vi "Begin.vi"(8 "error in":errorcluster) -> (0 "error out":errorcluster)   [LabVIEW 2014]
doc: "Called before other user functions, this VI is expected to open initial I/O refnums, load in file data, and do all program initialization. Notice that the <B>error out</B> terminal is simply used for data flow. Wiring it to other structures or subVIs ensures that this VI runs first."
uses:
  <vilib>/Rock Robotics/WPI/DriverStation/WPI_DriverStationRobotMode2.ctl
  <vilib>/Rock Robotics/WPI/Joystick/WPI_JoystickDeviceEnum.ctl
  <vilib>/Rock Robotics/SystemInterfaces/DIO/FPGA_DIOChannel.ctl
  <vilib>/Rock Robotics/WPI/Encoder/WPI_EncoderType.ctl
  <vilib>/Rock Robotics/WPI/Solenoid/WPI_SolenoidChannel.ctl
  <vilib>/Rock Robotics/SystemInterfaces/Typedef/FPGA_TypedefDigitalModule.ctl
  <vilib>/Rock Robotics/SystemInterfaces/Typedef/FPGA_TypedefAnalogModuleForGyro.ctl
  <vilib>/Rock Robotics/SystemInterfaces/AI/FPGA_AIGyroChannel.ctl
  <vilib>/Rock Robotics/WPI/SafetyOutput/WPI_SafetyOutputConfigMenu.ctl
  Robot Global Data.vi
  <vilib>/Rock Robotics/Network Tables/SD Write String Array.vi
  <vilib>/Rock Robotics/WPI/Counter/WPI_CounterDigitalInputToDigitalSource.vi
  <vilib>/Rock Robotics/WPI/Solenoid/WPI_SolenoidOpenDouble.vi
  <vilib>/Rock Robotics/WPI/Compressor/WPI_CompressorGetSetRefNum.vi
  <vilib>/Rock Robotics/WPI/MotorControl/WPI_MotorControlOpenCANTalonSRX.vi
  <vilib>/Rock Robotics/WPI/RobotDrive/WPI_RobotDriveOpen2MotorWithCANTalonSRX.vi
  <vilib>/Rock Robotics/SystemInterfaces/DIO/FPGA_DIOPWMChannel.ctl
  <vilib>/Rock Robotics/WPI/MotorControl/WPI_MotorControlOpen Talon.vi
  <vilib>/Rock Robotics/SystemInterfaces/i2clib/i2c_bus.ctl
  <vilib>/Rock Robotics/WPI/RobotDrive/WPI_RobotDriveOpen4MotorWithCANTalonSRX.vi
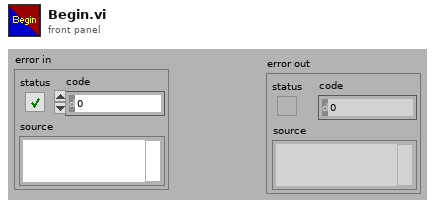
[diagram p1: front panel]
types:
  T1 = typedef "WPI_JoystickDeviceEnum.ctl" = enum16{"USB 0", "USB 1", "USB 2", "USB 3", "USB 4", "USB 5"}
  T2 = typedef "FPGA_DIOChannel.ctl" = enum8{"DIO 0", "DIO 1", "DIO 2", "DIO 3", "DIO 4", "DIO 5", "DIO 6", "DIO 7", "DIO 8", "DIO 9", "DIO MXP 0", "DIO MXP 1", "DIO MXP 2", "DIO MXP 3", "DIO MXP 4", "DIO MXP 5", "DIO MXP 6", "DIO MXP 7", "DIO MXP 8", "DIO MXP 9", "DIO MXP 10", "DIO MXP 11", "DIO MXP 12", "DIO MXP 13", "DIO MXP 14", "DIO MXP 15", "Invalid"}
  T3 = typedef "WPI_SolenoidChannel.ctl" = enum8{"Solenoid 0", "Solenoid 1", "Solenoid 2", "Solenoid 3", "Solenoid 4", "Solenoid 5", "Solenoid 6", "Solenoid 7", "Invalid"}
  T4 = typedef "FPGA_TypedefDigitalModule.ctl" = enum16{"Controller 1"}
  T5 = typedef "FPGA_AIGyroChannel.ctl" = enum8{"AI 0", "AI 1", "Invalid"}
  T6 = typedef "FPGA_TypedefAnalogModuleForGyro.ctl" = enum16{"Controller 1"}
  T7 = typedef "WPI_EncoderType.ctl" = enum16{"1x", "2x", "4x"}
  T8 = typedef "WPI_DriverStationRobotMode2.ctl" = enum16{"Autonomous Disabled", "Autonomous Enabled", "Teleop Disabled", "Teleop Enabled", "Disconnected", "Finish", "Test Disabled", "Test Enabled", "Emergency Stopped"}
  T9 = typedef "WPI_JoystickDevRef.ctl" = cluster{"Device":T1}
  T10 = typedef "WPI_CompressorDevRef.ctl" = cluster{"DevStatus":errorcluster, "Pneumatics Control Module":u8}
  T11 = typedef "WPI_SafetyOutputConfigMenu.ctl" = enum16{"Enable", "Disable"}
  T12 = typedef "WPI_RobotDriveDevRef.ctl" = cluster{"DevStatus":errorcluster, "Motors[]":T13[], "Square Inputs":bool, "Max Output":dbl}
  T13 = typedef "WPI_MotorControlDeviceRef.ctl" = cluster{"DeviceStatus":errorcluster, "Type":T14, "PWM":cluster{"Controller":T4, "PWM Channel":T15, "DeadBand":T16}, "CAN":cluster{"Device Number":u8, "Control Mode":T17, "Semaphore":T18, "Max Vout":dbl, "TalonSRX Control Mode":T19}, "Invert":bool, "TransformRef":T20, "InvTransformRef":T20}
  T14 = typedef "WPI_MotorControlType.ctl" = enum16{"PWM", "CAN", "CANTalonSRX"}
  T15 = typedef "FPGA_DIOPWMChannel.ctl" = enum8{"PWM 0", "PWM 1", "PWM 2", "PWM 3", "PWM 4", "PWM 5", "PWM 6", "PWM 7", "PWM 8", "PWM 9", "PWM MXP 0", "PWM MXP 1", "PWM MXP 2", "PWM MXP 3", "PWM MXP 4", "PWM MXP 5", "PWM MXP 6", "PWM MXP 7", "PWM MXP 8", "PWM MXP 9", "Invalid"}
  T16 = typedef "WPI_PWMDeadband.ctl" = cluster{"Name":string, "maxPositivePwm":i32, "minPositivePwm":i32, "centerPwm":i32, "maxNegativePwm":i32, "minNegativePwm":i32, "angularRange":u16}
  T17 = typedef "WPI_CANJaguar_ControlMode.ctl" = enum8{"Percent VBus", "Current", "Speed", "Position", "Voltage"}
  T18 = typedef "Semaphore RefNum" = refnum<k1>
  T19 = typedef "WPI_CANTalonSRX_APIControlMode.ctl" = enum8{"Percent VBus", "Speed", "Position", "Slave", "Unchanged / Invalid"}
  T20 = typedef "WPI_PWMTransform_ConPane.ctl" = refnum<vi>
  T21 = typedef "WPI_DigitalInputDevRef.ctl" = cluster{"DevStatus":errorcluster, "DIO Channel":T2, "Controller":T4}
  T22 = typedef "WPI_SolenoidDevRef.ctl" = cluster{"DevStatus":errorcluster, "Pneumatics Control Module":u8, "Forward Solenoid Channel":T3, "Reverse Solenoid Channel":T3}
  T23 = typedef "FPGA_CounterEncoderSourceConvertionLVSourceType.ctl" = cluster{"DevStatus":errorcluster, "AnalogTriggerMode?":bool, "DigitalMode":cluster{"Controller":T4, "DIO Channel":T24}, "AnalogTriggerMode":cluster{"AnalogTriggerIndex":T25, "OutputType":T26}}
  T24 = typedef "FPGA_DIODigitalSourceChannel.ctl" = enum8{"DIO 0", "DIO 1", "DIO 2", "DIO 3", "DIO 4", "DIO 5", "DIO 6", "DIO 7", "DIO 8", "DIO 9", "DIO MXP 0", "DIO MXP 1", "DIO MXP 2", "DIO MXP 3", "DIO MXP 4", "DIO MXP 5", "DIO MXP 6", "DIO MXP 7", "DIO MXP 8", "DIO MXP 9", "DIO MXP 10", "DIO MXP 11", "DIO MXP 12", "DIO MXP 13", "DIO MXP 14", "DIO MXP 15", "Disabled"}
  T25 = typedef "FPGA_AnalogTriggerIndex.ctl" = enum8{"Trig 0", "Trig 1", "Trig 2", "Trig 3", "Trig 4", "Trig 5", "Trig 6", "Trig 7", "Invalid"}
  T26 = typedef "FPGA_AnalogTriggerOutType.ctl" = enum16{"InWindow", "TriggerState", "Rising", "Falling"}
  T27 = typedef "WPI_EncoderDevRef.ctl" = cluster{"DevStatus":errorcluster, "EncoderIndex":T28, "CounterIndex":T29, "DistancePerCount":dbl, "Decoding Type":T7}
  T28 = typedef "FPGA_EncoderIdx.ctl" = enum8{"Enc 0", "Enc 1", "Enc 2", "Enc 3", "Enc 4", "Enc 5", "Enc 6", "Enc 7", "Invalid"}
  T29 = typedef "FPGA_CounterCtrSystemIndex.ctl" = enum8{"Ctr 0", "Ctr 1", "Ctr 2", "Ctr 3", "Ctr 4", "Ctr 5", "Ctr 6", "Ctr 7", "Invalid"}
  T30 = typedef "WPI_GyroDevRef.ctl" = cluster{"DevStatus":errorcluster, "Analog Module":T31, "Analog Channel":T32, "Offset":dbl, "Gain (VoltsPerDegree/Second)":dbl}
  T31 = typedef "FPGA_TypedefAnalogModule.ctl" = enum16{"Controller 1"}
  T32 = typedef "FPGA_AIChannel.ctl" = enum8{"AI 0", "AI 1", "AI 2", "AI 3", "AI MXP 0", "AI MXP 1", "AI MXP 2", "AI MXP 3", "Invalid"}
  T33 = typedef "i2c_bus.ctl" = enum16{"I2C On-Board", "I2C MXP", "Invalid"}
  T34 = typedef "WPI_ServoDeviceRef.ctl" = cluster{"DeviceStatus":errorcluster, "Controller":T4, "PWM Channel":T15, "DeadBand":T16}
  T35 = typedef "WPI_I2CDevRef.ctl" = cluster{"DevStatus":errorcluster, "Controller":T4, "Device Address":u8, "Handle":i32, "I2C Bus":T33}
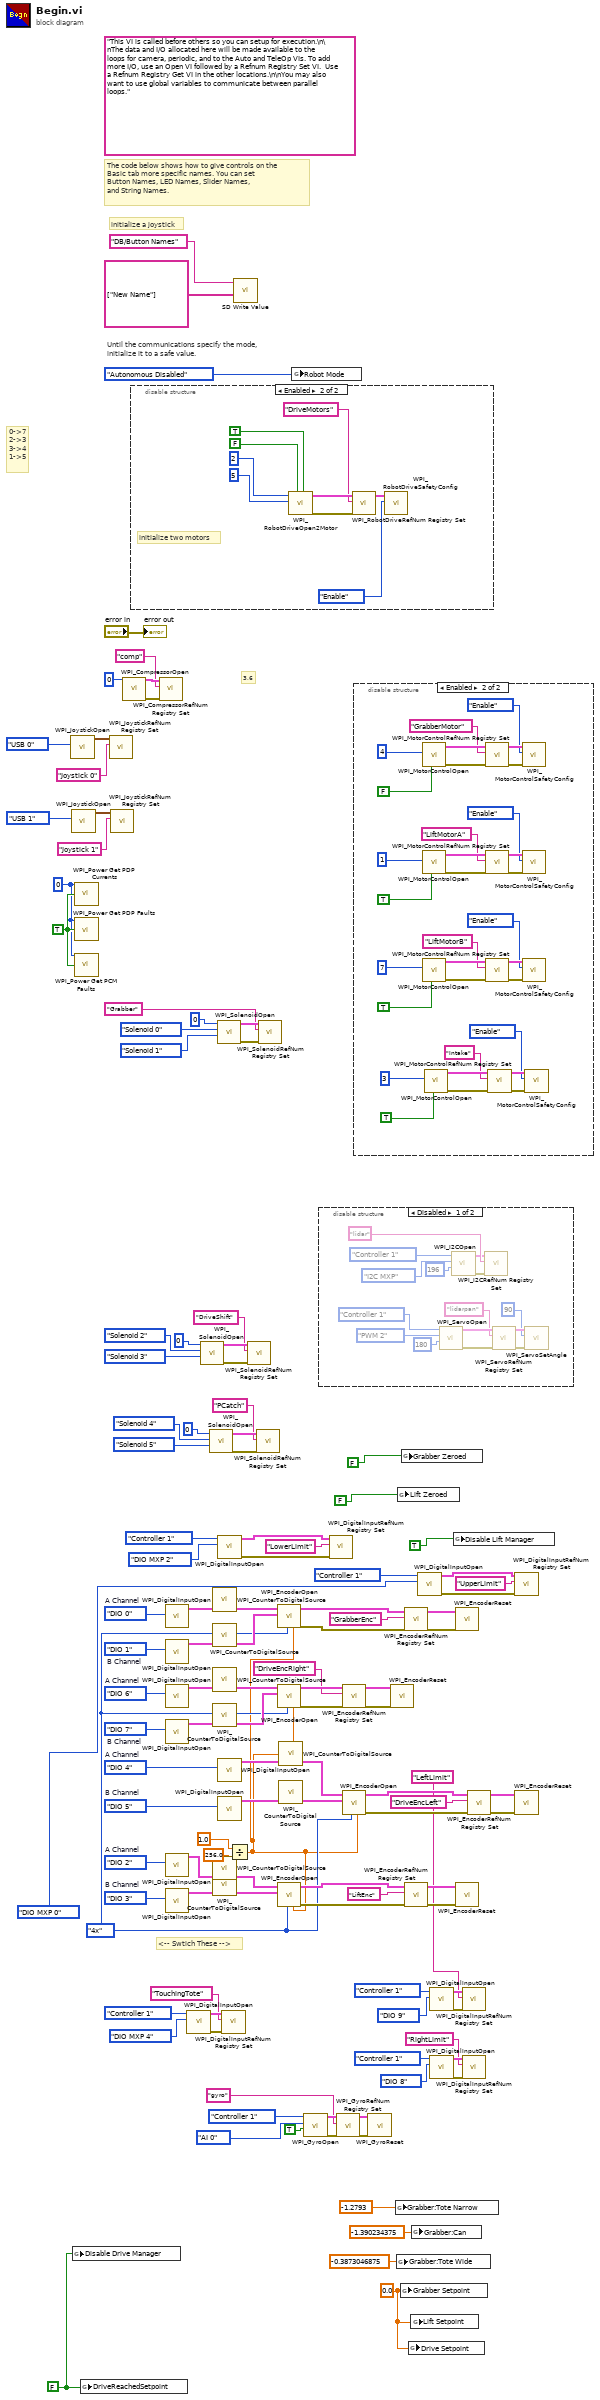
[diagram p0: block diagram]
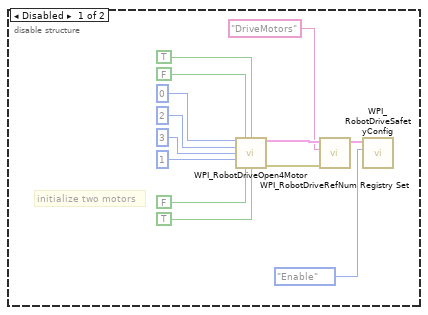
[diagram p2: hidden frame]
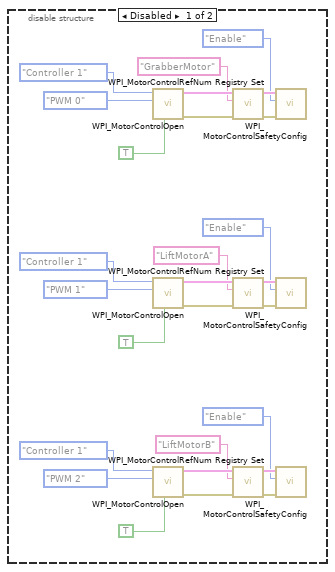
[diagram p3: hidden frame]
diagram:
  w1 = FALSE
  w2 = 0.0 ("Grabber Setpoint")
  w9 = u8 0 ("Power Distribution Panel (0)")
  w10 = TRUE ("Tare Currents?")
  w26 = FPGA_DIOChannel."DIO 7"  # B Channel
  w25 = FPGA_DIOChannel."DIO 6"  # A Channel
  w61 = FPGA_DIOChannel."DIO 5"  # B Channel
  w60 = FPGA_DIOChannel."DIO 4"  # A Channel
  w72 = FPGA_DIOChannel."DIO 1"  # B Channel
  w71 = FPGA_DIOChannel."DIO 0"  # A Channel
  w15 = WPI_EncoderType."4x" ("Decoding Type")
  w116 = FPGA_DIOChannel."DIO 3"  # B Channel
  w115 = FPGA_DIOChannel."DIO 2"  # A Channel
  (unwired) "This VI is called before others so you can setup for execution.\n\nThe data and I/O allocated here will be made available to the loops for camera, periodic, and to the Auto and TeleOp VIs. To add more I/O, use an Open VI followed by a Refnum Registry Set VI.  Use a Refnum Registry Get VI in the other locations.\n\nYou may also want to use global variables to communicate between parallel loops."
  # "3,6"
  # "0->7\n2->3\n3->4\n1->5"
  # "<-- Swtich These -->"
  # "The code below shows how to give controls on the\nBasic tab more specific names. You can set\nButton Names, LED Names, Slider Names,\nand String Names."
  # "initialize a joystick"
  # "Until the communications specify the mode,\ninitialize it to a safe value."
  n1 = call <vilib>:"WPI_JoystickOpen.vi"("JoystickDevice"=WPI_JoystickDeviceEnum."USB 0") -> ("JoystickDevRef"=w121:T9)  [unwired: 10 in]
  n2 = call <vilib>:"WPI_JoystickOpen.vi"("JoystickDevice"=WPI_JoystickDeviceEnum."USB 1") -> ("JoystickDevRef"=w12:T9)  [unwired: 10 in]
  n3 = global write "Robot Global Data.vi" "Disable Drive Manager"(w1) -> ()
  n4 = call <vilib>:"WPI_Power Get PDP Currents.vi"("Power Distribution Panel (0)"=w9, "Tare Currents?"=w10) -> ()  [unwired: 11 in, 3 out]
  n5 = call <vilib>:"WPI_Power Get PDP Faults.vi"("Power Distribution Panel (0)"=w9, "Clear Sticky Faults"=w10) -> ()  [unwired: 9 in, 5 out]
  n6 = call <vilib>:"WPI_Power Get PCM Faults.vi"("Pneumatics Control Module (0)"=w9, "Clear Sticky Faults"=w10) -> ()  [unwired: 10 in, 4 out]
  n7 = global write "Robot Global Data.vi" "DriveReachedSetpoint"(w1) -> ()
  n8 = call <vilib>:"WPI_JoystickRefNum Registry Set.vi"("refnum name"="Joystick 0", "JoystickDevRef"=w121) -> ()  [unwired: 8 in, 2 out]
  n9 = call <vilib>:"WPI_JoystickRefNum Registry Set.vi"("refnum name"="Joystick 1", "JoystickDevRef"=w12) -> ()  [unwired: 8 in, 2 out]
  n10 = call <vilib>:"WPI_CompressorOpen.vi"("Pneumatics Control Module (0)"=u8 0) -> ("CompressorDevRef"=w74:T10, "error out"=w75:errorcluster)  [unwired: 13 in]
  n11 = disable-structure shown="Enabled" {
    frame Disabled {
      # "initialize two motors"
      n12 = call-poly <vilib>:"WPI_RobotDriveOpen4Motor.vi"("Rear Left Motor"=u8 0, "Rear Left Motor Inverted"=FALSE, "Rear Right Motor Inverted"=TRUE, "Rear Right Motor"=u8 2, "Front Left Motor"=u8 3, "Front Right Motor"=u8 1, "Front Left Motor Inverted"=FALSE, "Front Right Motor Inverted"=TRUE) -> ("RobotDriveDevRef"=w136:T12, "error out"=w134:errorcluster)  [unwired: 6 in]
      n13 = call <vilib>:"WPI_RobotDriveRefNum Registry Set.vi"("error in (no error)"=w134, "refnum name"="DriveMotors", "RobotDriveDevRef"=w136) -> ("RobotDriveDevRef"=w133:T12)  [unwired: 8 out]
      n14 = call <vilib>:"WPI_RobotDriveSafetyConfig.vi"("mode"=WPI_SafetyOutputConfigMenu."Enable", "RobotDriveDevRef"=w133) -> ()  [unwired: 8 in, 2 out]
    }
    frame Enabled {
      # "initialize two motors"
      n15 = call-poly <vilib>:"WPI_RobotDriveOpen2Motor.vi"("Right Motor Inverted"=TRUE ("Rear Right Motor Inverted"), "Left Motor Inverted"=FALSE ("Rear Left Motor Inverted"), "Right Motor"=u8 5 ("Rear Right Motor"), "Left Motor"=u8 2 ("Rear Left Motor")) -> ("error out"=w144:errorcluster, "RobotDriveDevRef"=w145:T12)  [unwired: 6 in]
      n16 = call <vilib>:"WPI_RobotDriveRefNum Registry Set.vi"("error in (no error)"=w144, "refnum name"="DriveMotors", "RobotDriveDevRef"=w145) -> ("RobotDriveDevRef"=w143:T12)  [unwired: 8 out]
      n17 = call <vilib>:"WPI_RobotDriveSafetyConfig.vi"("mode"=WPI_SafetyOutputConfigMenu."Enable", "RobotDriveDevRef"=w143) -> ()  [unwired: 8 in, 2 out]
    }
  }
  n18 = call <vilib>:"WPI_CompressorRefNum Registry Set.vi"("error in (no error)"=w75, "refnum name"="comp", "CompressorDevRef"=w74) -> ()  [unwired: 7 in, 2 out]
  n19 = call <vilib>:"WPI_DigitalInputOpen.vi"("DIO Channel"=w71) -> ("DigitalInputDevRef"=w68:T21)  [unwired: 2 in, 8 out]
  n20 = call <vilib>:"WPI_DigitalInputOpen.vi"("DIO Channel"=w72) -> ("DigitalInputDevRef"=w69:T21)  [unwired: 2 in, 8 out]
  n21 = call <vilib>:"WPI_DigitalInputOpen.vi"("DIO Channel"=w25) -> ("DigitalInputDevRef"=w22:T21)  [unwired: 2 in, 8 out]
  n22 = call <vilib>:"WPI_DigitalInputOpen.vi"("DIO Channel"=w26) -> ("DigitalInputDevRef"=w23:T21)  [unwired: 2 in, 8 out]
  n23 = call <vilib>:"WPI_DigitalInputOpen.vi"("DIO Channel"=w115) -> ("DigitalInputDevRef"=w112:T21)  [unwired: 2 in, 8 out]
  n24 = call <vilib>:"WPI_DigitalInputOpen.vi"("DIO Channel"=w116) -> ("DigitalInputDevRef"=w113:T21)  [unwired: 2 in, 8 out]
  n25 = call <vilib>:"WPI_DigitalInputOpen.vi"("DIO Channel"=FPGA_DIOChannel."DIO MXP 4", "Controller"=FPGA_TypedefDigitalModule."Controller 1") -> ("error out"=w79:errorcluster, "DigitalInputDevRef"=w78:T21)  [unwired: 8 in]
  n26 = call-poly <vilib>:"WPI_SolenoidOpen.vi"("Reverse Solenoid Channel"=WPI_SolenoidChannel."Solenoid 3", "Forward Solenoid Channel"=WPI_SolenoidChannel."Solenoid 2" ("Solenoid Channel"), "Pneumatics Control Module (0)"=u8 0) -> ("error out"=w94:errorcluster, "SolenoidDevRef"=w93:T22)  [unwired: 7 in]
  n27 = call-poly <vilib>:"WPI_SolenoidOpen.vi"("Reverse Solenoid Channel"=WPI_SolenoidChannel."Solenoid 5", "Forward Solenoid Channel"=WPI_SolenoidChannel."Solenoid 4" ("Solenoid Channel"), "Pneumatics Control Module (0)"=u8 0) -> ("error out"=w29:errorcluster, "SolenoidDevRef"=w28:T22)  [unwired: 7 in]
  n28 = call-poly <vilib>:"WPI_CounterToDigitalSource.vi"("DigitalInputDevRef"=w68) -> ("Digital Source"=w67:T23)  [unwired: 6 out]
  n29 = call-poly <vilib>:"WPI_CounterToDigitalSource.vi"("DigitalInputDevRef"=w69) -> ("Digital Source"=w70:T23)  [unwired: 6 out]
  n30 = call-poly <vilib>:"WPI_CounterToDigitalSource.vi"("DigitalInputDevRef"=w22) -> ("Digital Source"=w21:T23)  [unwired: 6 out]
  n31 = call-poly <vilib>:"WPI_CounterToDigitalSource.vi"("DigitalInputDevRef"=w23) -> ("Digital Source"=w24:T23)  [unwired: 6 out]
  n32 = call-poly <vilib>:"WPI_CounterToDigitalSource.vi"("DigitalInputDevRef"=w112) -> ("Digital Source"=w111:T23)  [unwired: 6 out]
  n33 = call-poly <vilib>:"WPI_CounterToDigitalSource.vi"("DigitalInputDevRef"=w113) -> ("Digital Source"=w114:T23)  [unwired: 6 out]
  n34 = call-poly <vilib>:"WPI_SolenoidOpen.vi"("Reverse Solenoid Channel"=WPI_SolenoidChannel."Solenoid 1", "Forward Solenoid Channel"=WPI_SolenoidChannel."Solenoid 0" ("Solenoid Channel"), "Pneumatics Control Module (0)"=u8 0) -> ("error out"=w100:errorcluster, "SolenoidDevRef"=w99:T22)  [unwired: 7 in]
  n35 = call <vilib>:"WPI_DigitalInputOpen.vi"("DIO Channel"=FPGA_DIOChannel."DIO MXP 2", "Controller"=FPGA_TypedefDigitalModule."Controller 1") -> ("error out"=w89:errorcluster, "DigitalInputDevRef"=w88:T21)  [unwired: 8 in]
  n36 = call <vilib>:"WPI_DigitalInputOpen.vi"("DIO Channel"=w60) -> ("DigitalInputDevRef"=w57:T21)  [unwired: 2 in, 8 out]
  n37 = call <vilib>:"WPI_DigitalInputOpen.vi"("DIO Channel"=w61) -> ("DigitalInputDevRef"=w58:T21)  [unwired: 2 in, 8 out]
  n38 = call <vilib>:"WPI_DigitalInputRefNum Registry Set.vi"("error in (no error)"=w79, "refnum name"="TouchingTote", "DigitalInputDevRef"=w78) -> ()  [unwired: 7 in, 2 out]
  n39 = Divide(x=1.0 ("DistancePerCount"), y=256.0) -> (x/y=w14:dbl)
  n40 = call-poly <vilib>:"SD Write Value.vi"("String Array"=string[] ["New Name"], "Name"="DB/Button Names") -> ()  [unwired: 8 in, 2 out]
  n41 = call <vilib>:"WPI_SolenoidRefNum Registry Set.vi"("error in (no error)"=w94, "refnum name"="DriveShift", "SolenoidDevRef"=w93) -> ()  [unwired: 7 in, 2 out]
  n42 = call <vilib>:"WPI_SolenoidRefNum Registry Set.vi"("error in (no error)"=w29, "refnum name"="PCatch", "SolenoidDevRef"=w28) -> ()  [unwired: 7 in, 2 out]
  n43 = call <vilib>:"WPI_SolenoidRefNum Registry Set.vi"("error in (no error)"=w100, "refnum name"="Grabber", "SolenoidDevRef"=w99) -> ()  [unwired: 7 in, 2 out]
  n44 = call <vilib>:"WPI_EncoderOpen.vi"("DistancePerCount"=w14, "Decoding Type"=w15, "BSource"=w70, "ASource"=w67) -> ("error out"=w66:errorcluster, "EncoderDevRef"=w65:T27)  [unwired: 4 in, 2 out]
  n45 = call <vilib>:"WPI_EncoderOpen.vi"("DistancePerCount"=w14, "Decoding Type"=w15, "BSource"=w24, "ASource"=w21) -> ("error out"=w20:errorcluster, "EncoderDevRef"=w19:T27)  [unwired: 4 in, 2 out]
  n46 = call <vilib>:"WPI_EncoderOpen.vi"("DistancePerCount"=w14, "Decoding Type"=w15, "BSource"=w114, "ASource"=w111) -> ("error out"=w110:errorcluster, "EncoderDevRef"=w109:T27)  [unwired: 4 in, 2 out]
  n47 = call-poly <vilib>:"WPI_CounterToDigitalSource.vi"("DigitalInputDevRef"=w57) -> ("Digital Source"=w56:T23)  [unwired: 6 out]
  n48 = call-poly <vilib>:"WPI_CounterToDigitalSource.vi"("DigitalInputDevRef"=w58) -> ("Digital Source"=w59:T23)  [unwired: 6 out]
  n49 = global write "Robot Global Data.vi" "Robot Mode"(WPI_DriverStationRobotMode2."Autonomous Disabled" ("Robot Mode")) -> ()
  n50 = call <vilib>:"WPI_GyroOpen.vi"("Calibrate On Open"=TRUE, "Analog Channel"=FPGA_AIGyroChannel."AI 0", "Controller"=FPGA_TypedefAnalogModuleForGyro."Controller 1") -> ("error out"=w47:errorcluster, "GyroDevRef"=w46:T30)  [unwired: 6 in, 1 out]
  n51 = disable-structure shown="Disabled" {
    frame Disabled {
      n52 = call <vilib>:"WPI_ServoOpen.vi"("Angular Range"=u16 180, "PWM Channel"=FPGA_DIOPWMChannel."PWM 2", "Controller"=FPGA_TypedefDigitalModule."Controller 1") -> ("error out"=w153:errorcluster, "ServoDeviceRef"=w154:T34)  [unwired: 7 in]
      n53 = call <vilib>:"WPI_I2COpen.vi"("Device Address"=u8 196, "I2C Bus"=i2c_bus."I2C MXP", "Controller"=FPGA_TypedefDigitalModule."Controller 1") -> ("error out"=w147:errorcluster, "I2CDevRef"=w148:T35)  [unwired: 7 in]
      n54 = call <vilib>:"WPI_I2CRefNum Registry Set.vi"("error in (no error)"=w147, "refnum name"="lidar", "I2CDevRef"=w148) -> ()  [unwired: 7 in, 2 out]
      n55 = call <vilib>:"WPI_ServoRefNum Registry Set.vi"("error in (no error)"=w153, "refnum name"="lidarpan", "ServoDeviceRef"=w154) -> ("error out"=w151:errorcluster, "ServoDeviceRef"=w150:T34)  [unwired: 7 in]
      n56 = call <vilib>:"WPI_ServoSetAngle.vi"("error in (no error)"=w151, "Angle"=90, "ServoDeviceRef"=w150) -> ()  [unwired: 7 in, 2 out]
    }
    frame Enabled {
    }
  }
  n57 = call <vilib>:"WPI_DigitalInputRefNum Registry Set.vi"("error in (no error)"=w89, "refnum name"="LowerLimit", "DigitalInputDevRef"=w88) -> ()  [unwired: 7 in, 2 out]
  n58 = call <vilib>:"WPI_GyroRefNum Registry Set.vi"("error in (no error)"=w47, "refnum name"="gyro", "GyroDevRef"=w46) -> ("error out"=w44:errorcluster, "GyroDevRef"=w43:T30)  [unwired: 7 in]
  n59 = call <vilib>:"WPI_EncoderRefNum Registry Set.vi"("error in (no error)"=w20, "refnum name"="DriveEncRight", "EncoderDevRef"=w19) -> ("error out"=w17:errorcluster, "EncoderDevRef"=w18:T27)  [unwired: 7 in]
  n60 = call <vilib>:"WPI_EncoderOpen.vi"("DistancePerCount"=w14, "Decoding Type"=w15, "BSource"=w59, "ASource"=w56) -> ("error out"=w55:errorcluster, "EncoderDevRef"=w54:T27)  [unwired: 4 in, 2 out]
  n61 = disable-structure shown="Enabled" {
    frame Disabled {
      n62 = call-poly <vilib>:"WPI_MotorControlOpen.vi"("Invert"=TRUE, "PWM Channel"=FPGA_DIOPWMChannel."PWM 0", "Controller"=FPGA_TypedefDigitalModule."Controller 1") -> ("error out"=w167:errorcluster, "MotorControlDeviceRef"=w166:T13)  [unwired: 7 in]
      n63 = call-poly <vilib>:"WPI_MotorControlOpen.vi"("Invert"=TRUE, "PWM Channel"=FPGA_DIOPWMChannel."PWM 1", "Controller"=FPGA_TypedefDigitalModule."Controller 1") -> ("error out"=w179:errorcluster, "MotorControlDeviceRef"=w180:T13)  [unwired: 7 in]
      n64 = call-poly <vilib>:"WPI_MotorControlOpen.vi"("Invert"=TRUE, "PWM Channel"=FPGA_DIOPWMChannel."PWM 2", "Controller"=FPGA_TypedefDigitalModule."Controller 1") -> ("error out"=w182:errorcluster, "MotorControlDeviceRef"=w181:T13)  [unwired: 7 in]
      n65 = call <vilib>:"WPI_MotorControlRefNum Registry Set.vi"("error in (no error)"=w167, "refnum name"="GrabberMotor", "MotorControlDevRef"=w166) -> ("error out"=w163:errorcluster, "MotorControlDevRef"=w162:T13)  [unwired: 7 in]
      n66 = call <vilib>:"WPI_MotorControlRefNum Registry Set.vi"("error in (no error)"=w179, "refnum name"="LiftMotorA", "MotorControlDevRef"=w180) -> ("error out"=w173:errorcluster, "MotorControlDevRef"=w172:T13)  [unwired: 7 in]
      n67 = call <vilib>:"WPI_MotorControlRefNum Registry Set.vi"("error in (no error)"=w182, "refnum name"="LiftMotorB", "MotorControlDevRef"=w181) -> ("error out"=w175:errorcluster, "MotorControlDevRef"=w174:T13)  [unwired: 7 in]
      n68 = call <vilib>:"WPI_MotorControlSafetyConfig.vi"("error in (no error)"=w163, "mode"=WPI_SafetyOutputConfigMenu."Enable", "MotorControlDevRef"=w162) -> ()  [unwired: 7 in, 2 out]
      n69 = call <vilib>:"WPI_MotorControlSafetyConfig.vi"("error in (no error)"=w173, "mode"=WPI_SafetyOutputConfigMenu."Enable", "MotorControlDevRef"=w172) -> ()  [unwired: 7 in, 2 out]
      n70 = call <vilib>:"WPI_MotorControlSafetyConfig.vi"("error in (no error)"=w175, "mode"=WPI_SafetyOutputConfigMenu."Enable", "MotorControlDevRef"=w174) -> ()  [unwired: 7 in, 2 out]
    }
    frame Enabled {
      n71 = call-poly <vilib>:"WPI_MotorControlOpen.vi"("Invert"=FALSE, "Device Number"=u8 4) -> ("error out"=w205:errorcluster, "MotorControlDeviceRef"=w204:T13)  [unwired: 8 in]
      n72 = call-poly <vilib>:"WPI_MotorControlOpen.vi"("Invert"=TRUE, "Device Number"=u8 1) -> ("error out"=w215:errorcluster, "MotorControlDeviceRef"=w216:T13)  [unwired: 8 in]
      n73 = call-poly <vilib>:"WPI_MotorControlOpen.vi"("Invert"=TRUE, "Device Number"=u8 7) -> ("error out"=w218:errorcluster, "MotorControlDeviceRef"=w217:T13)  [unwired: 8 in]
      n74 = call-poly <vilib>:"WPI_MotorControlOpen.vi"("Invert"=TRUE, "Device Number"=u8 3) -> ("error out"=w195:errorcluster, "MotorControlDeviceRef"=w194:T13)  [unwired: 8 in]
      n75 = call <vilib>:"WPI_MotorControlRefNum Registry Set.vi"("error in (no error)"=w205, "refnum name"="GrabberMotor", "MotorControlDevRef"=w204) -> ("error out"=w201:errorcluster, "MotorControlDevRef"=w200:T13)  [unwired: 7 in]
      n76 = call <vilib>:"WPI_MotorControlRefNum Registry Set.vi"("error in (no error)"=w215, "refnum name"="LiftMotorA", "MotorControlDevRef"=w216) -> ("error out"=w209:errorcluster, "MotorControlDevRef"=w208:T13)  [unwired: 7 in]
      n77 = call <vilib>:"WPI_MotorControlRefNum Registry Set.vi"("error in (no error)"=w218, "refnum name"="LiftMotorB", "MotorControlDevRef"=w217) -> ("error out"=w211:errorcluster, "MotorControlDevRef"=w210:T13)  [unwired: 7 in]
      n78 = call <vilib>:"WPI_MotorControlRefNum Registry Set.vi"("error in (no error)"=w195, "refnum name"="Intake", "MotorControlDevRef"=w194) -> ("error out"=w191:errorcluster, "MotorControlDevRef"=w190:T13)  [unwired: 7 in]
      n79 = call <vilib>:"WPI_MotorControlSafetyConfig.vi"("error in (no error)"=w201, "mode"=WPI_SafetyOutputConfigMenu."Enable", "MotorControlDevRef"=w200) -> ()  [unwired: 7 in, 2 out]
      n80 = call <vilib>:"WPI_MotorControlSafetyConfig.vi"("error in (no error)"=w209, "mode"=WPI_SafetyOutputConfigMenu."Enable", "MotorControlDevRef"=w208) -> ()  [unwired: 7 in, 2 out]
      n81 = call <vilib>:"WPI_MotorControlSafetyConfig.vi"("error in (no error)"=w211, "mode"=WPI_SafetyOutputConfigMenu."Enable", "MotorControlDevRef"=w210) -> ()  [unwired: 7 in, 2 out]
      n82 = call <vilib>:"WPI_MotorControlSafetyConfig.vi"("error in (no error)"=w191, "mode"=WPI_SafetyOutputConfigMenu."Enable", "MotorControlDevRef"=w190) -> ()  [unwired: 7 in, 2 out]
    }
  }
  n83 = call <vilib>:"WPI_GyroReset.vi"("error in (no error)"=w44, "GyroDevRef"=w43) -> ()  [unwired: 8 in, 2 out]
  n84 = call <vilib>:"WPI_EncoderReset.vi"("error in (no error)"=w17, "EncoderDevRef"=w18) -> ()  [unwired: 8 in, 2 out]
  n85 = global write "Robot Global Data.vi" "Grabber:Tote Narrow"(-1.2793) -> ()
  n86 = global write "Robot Global Data.vi" "Grabber:Tote Wide"(-0.3873046875 ("Grabber:Tote Wide")) -> ()
  n87 = global write "Robot Global Data.vi" "Lift Zeroed"(FALSE) -> ()
  n88 = global write "Robot Global Data.vi" "Grabber Setpoint"(w2) -> ()
  n89 = global write "Robot Global Data.vi" "Grabber Zeroed"(FALSE) -> ()
  n90 = call <vilib>:"WPI_EncoderRefNum Registry Set.vi"("error in (no error)"=w66, "refnum name"="GrabberEnc", "EncoderDevRef"=w65) -> ("error out"=w63:errorcluster, "EncoderDevRef"=w64:T27)  [unwired: 7 in]
  n91 = call <vilib>:"WPI_EncoderRefNum Registry Set.vi"("error in (no error)"=w110, "refnum name"="LiftEnc", "EncoderDevRef"=w109) -> ("error out"=w107:errorcluster, "EncoderDevRef"=w108:T27)  [unwired: 7 in]
  n92 = global write "Robot Global Data.vi" "Drive Setpoint"(w2) -> ()
  n93 = global write "Robot Global Data.vi" "Lift Setpoint"(w2) -> ()
  n94 = global write "Robot Global Data.vi" "Grabber:Can"(-1.390234375 ("Grabber:Can")) -> ()
  n95 = call <vilib>:"WPI_DigitalInputOpen.vi"("DIO Channel"=FPGA_DIOChannel."DIO MXP 0", "Controller"=FPGA_TypedefDigitalModule."Controller 1") -> ("error out"=w84:errorcluster, "DigitalInputDevRef"=w83:T21)  [unwired: 8 in]
  n96 = call <vilib>:"WPI_DigitalInputOpen.vi"("DIO Channel"=FPGA_DIOChannel."DIO 9", "Controller"=FPGA_TypedefDigitalModule."Controller 1") -> ("error out"=w40:errorcluster, "DigitalInputDevRef"=w39:T21)  [unwired: 8 in]
  n97 = call <vilib>:"WPI_DigitalInputOpen.vi"("DIO Channel"=FPGA_DIOChannel."DIO 8", "Controller"=FPGA_TypedefDigitalModule."Controller 1") -> ("error out"=w35:errorcluster, "DigitalInputDevRef"=w34:T21)  [unwired: 8 in]
  n98 = global write "Robot Global Data.vi" "Disable Lift Manager"(TRUE) -> ()
  n99 = call <vilib>:"WPI_EncoderReset.vi"("error in (no error)"=w63, "EncoderDevRef"=w64) -> ()  [unwired: 8 in, 2 out]
  n100 = call <vilib>:"WPI_EncoderReset.vi"("error in (no error)"=w107, "EncoderDevRef"=w108) -> ()  [unwired: 8 in, 2 out]
  n101 = call <vilib>:"WPI_DigitalInputRefNum Registry Set.vi"("error in (no error)"=w40, "refnum name"="LeftLimit", "DigitalInputDevRef"=w39) -> ()  [unwired: 7 in, 2 out]
  n102 = call <vilib>:"WPI_DigitalInputRefNum Registry Set.vi"("error in (no error)"=w35, "refnum name"="RightLimit", "DigitalInputDevRef"=w34) -> ()  [unwired: 7 in, 2 out]
  n103 = call <vilib>:"WPI_EncoderRefNum Registry Set.vi"("error in (no error)"=w55, "refnum name"="DriveEncLeft", "EncoderDevRef"=w54) -> ("error out"=w52:errorcluster, "EncoderDevRef"=w53:T27)  [unwired: 7 in]
  n104 = call <vilib>:"WPI_DigitalInputRefNum Registry Set.vi"("error in (no error)"=w84, "refnum name"="UpperLimit", "DigitalInputDevRef"=w83) -> ()  [unwired: 7 in, 2 out]
  n105 = call <vilib>:"WPI_EncoderReset.vi"("error in (no error)"=w52, "EncoderDevRef"=w53) -> ()  [unwired: 8 in, 2 out]
  "error out" <- "error in"
